vi "ExImageFileToSpreadsheet.vi"() -> ()   [LabVIEW 2010]
uses:
  <vilib>/Utility/file.llb/Write To Spreadsheet File (DBL).vi
panel:
  in  "2d Array Spreadsheet File Name (put in .xls on filename)":path
  in  "1d Array Spreadsheet File Name (put in .xls on filename)":path
  out "Test 2d Array":sgl[][](array[numeric]) format="%.2f"
  out "Test 1d array":sgl[](array[numeric]) format="%.2f"
  out "Pixel Value u16":u16
  out "Pixel Value i32":i32
  out "Pixel Value f32":sgl format="%.2f"
  out "error out":errorcluster
  in  "error in (no error)":errorcluster
  # "NOTICE\n\nTHIS VI REQUIRES THAT THE TOOLKIT\nBE UNLOADED BY RUNNING THE\n VI EXCLOSEGLOBALCAM.VI\n BEFORE LEAVING LABVIEW."
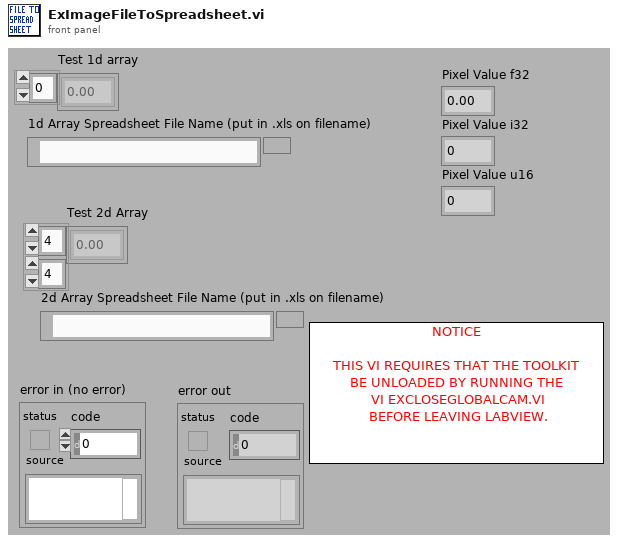
[diagram p1: front panel]
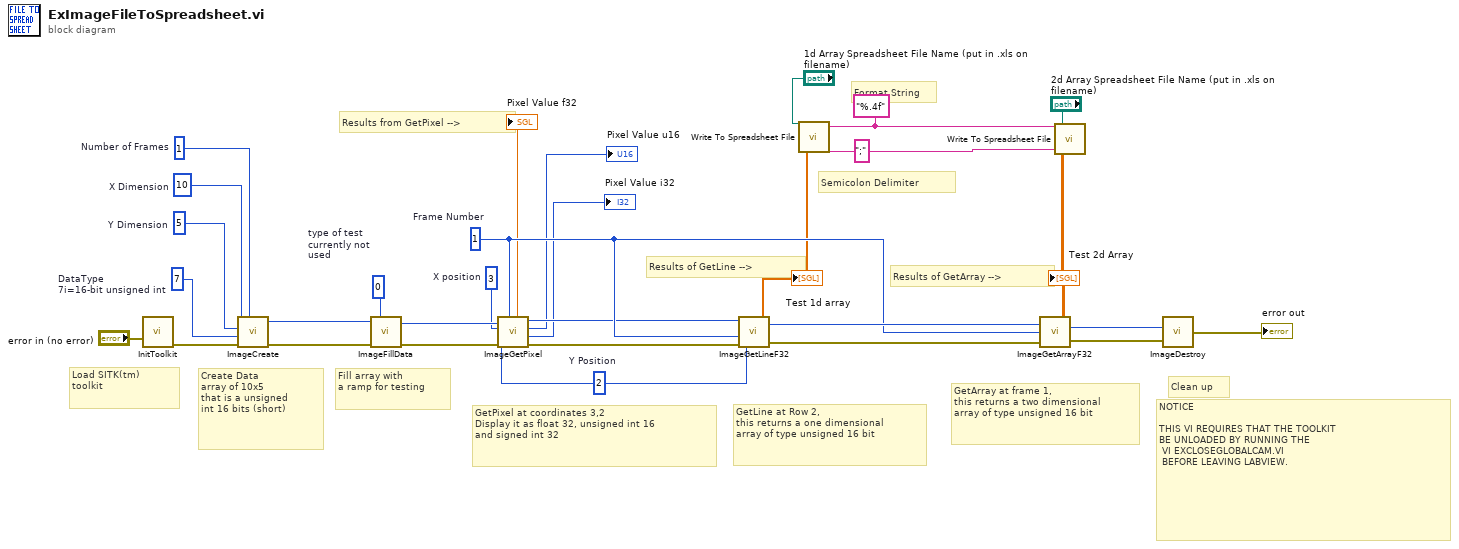
[diagram p0: block diagram]
diagram:
  w2 = ";"
  w3 = "%.4f"
  w13 = 1  # Frame Number
  w16 = 2  # Y Position
  w17 = 3  # X position
  w19 = 0  # type of test currently not used
  w21 = 1  # Number of Frames
  w22 = 10  # X Dimension
  w23 = 5  # Y Dimension
  w24 = 7  # DataType  7i=16-bit unsigned int
  # "NOTICE\n\nTHIS VI REQUIRES THAT THE TOOLKIT\nBE UNLOADED BY RUNNING THE\n VI EXCLOSEGLOBALCAM.VI\n BEFORE LEAVING LABVIEW."
  # "Format String"
  # "Semicolon Delimiter"
  # "Clean up"
  # "Results of GetArray -->"
  # "GetArray at frame 1,\nthis returns a two dimensional\narray of type unsigned 16 bit"
  # "GetLine at Row 2,\nthis returns a one dimensional\narray of type unsigned 16 bit"
  # "Results of GetLine -->"
  # "GetPixel at coordinates 3,2\nDisplay it as float 32, unsigned int 16\nand signed int 32"
  # "Results from GetPixel -->"
  # "Fill array with \na ramp for testing"
  # "Create Data\narray of 10x5\nthat is a unsigned \nint 16 bits (short)"
  # "Load SITK(tm) \ntoolkit"
  n1 = call <userlib>:"InitToolkit.vi"("error in"="error in (no error)") -> ("error out"=w30:errorcluster)
  n2 = call <userlib>:"ImageCreate.vi"("X dimension"=w22, "Y dimension"=w23, "Data Type"=w24, "error in"=w30, "Number Of Frames"=w21) -> ("Image Handle"=w20:u32, "error out"=w28:errorcluster)
  n3 = call <userlib>:"ImageFillData.vi"("error in"=w28, "Type of Test"=w19, "Image Handle"=w20) -> ("error out"=w27:errorcluster, "Image Handle"=w18:u32)
  n4 = call <userlib>:"ImageGetPixel.vi"("Z position"=w13, "error in"=w27, "Y position"=w16, "X position"=w17, "Data Handle"=w18) -> ("error out"=w11:errorcluster, "Pixel Value i32"=→"Pixel Value i32":i32, "Pixel Value u16"=→"Pixel Value u16":u16, "Data Handle"=w12:u32, "Pixel Value f32"=→"Pixel Value f32":sgl)
  n5 = call <userlib>:"ImageGetLineF32.vi"("error in"=w11, "Z Position"=w13, "Y Position"=w16, "Data Handle"=w12) -> ("error out"=w26:errorcluster, "Array F32"=w7:sgl[], "Data Handle"=w15:u32)
  "Test 1d array" <- w7
  n6 = call-poly <vilib>:"Write To Spreadsheet File.vi"("delimiter (\\t)"=w2, "format (%.3f)"=w3, "1D data"=w7, "file path (dialog if empty)"="1d Array Spreadsheet File Name (put in .xls on filename)") -> ()  [unwired: 4 in, 1 out]
  n7 = call <userlib>:"ImageGetArrayF32.vi"("error in"=w26, "Z position"=w13, "Image Handle"=w15) -> ("error out"=w25:errorcluster, "Array Float 32"=w6:sgl[][], "Image Handle"=w14:u32)
  "Test 2d Array" <- w6
  n8 = call-poly <vilib>:"Write To Spreadsheet File.vi"("delimiter (\\t)"=w2, "format (%.3f)"=w3, "2D data"=w6, "file path (dialog if empty)"="2d Array Spreadsheet File Name (put in .xls on filename)") -> ()  [unwired: 4 in, 1 out]
  n9 = call <userlib>:"ImageDestroy.vi"("error in"=w25, "Data handle"=w14) -> ("error out"=→"error out":errorcluster)
